vi "SR830 Read Channels.vi"(8 "error in (no error)":errorcluster caption="Error in (no error)", 10 "830?":bool, 11 "VISA Resource Name":refnum<visa-resource-name>) -> (0 "error out":errorcluster caption="Error", 1 "output2":dbl format="%#_12g", 2 "output1":dbl format="%#_12g", 3 "VISA resource name out":refnum<visa-resource-name>)   [LabVIEW 2017, in "SR830.lvlib"]
doc: "Reads the values currently displayed on the front panel of the lock-in detector."
uses:
  SR830.lvlib
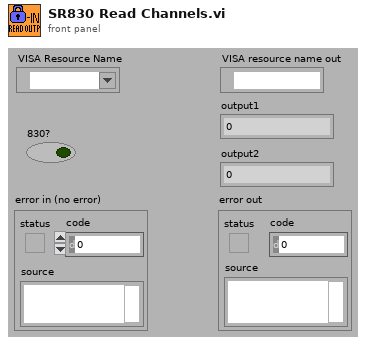
[diagram p1: front panel]
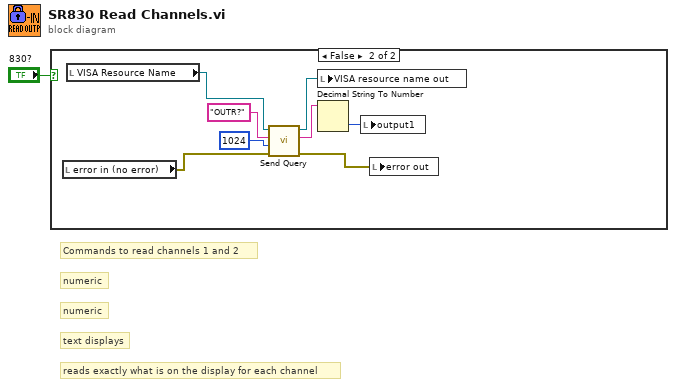
[diagram p0: block diagram]
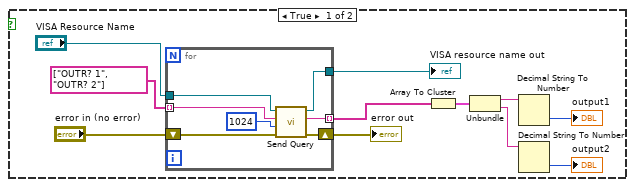
[diagram p2: hidden frame]
diagram:
  # "Commands to read channels 1 and 2"
  # "numeric"
  # "numeric"
  # "text displays"
  # "reads exactly what is on the display for each channel"
  n1 = case shown="False" "830?" {
    frame True {
      n2 = for {
        tunnel: [w15] -> w9 mode=indexing
        shift-right: [w14] -> w12
        shift-left: "error in (no error)" -> [w19]
        tunnel: "VISA Resource Name" -> [w16]
        tunnel: string[] ["OUTR? 1", "OUTR? 2"] -> [w17] mode=indexing
        tunnel: [w13] -> w6
        n3 = call "Send Query.vi"("error in (no error)"=w19, "Bytes Count"=1024, "write buffer"=w17, "VISA resource name"=w16) -> ("error out"=w14:errorcluster, "read buffer"=w15:string, "VISA resource name out"=w13:refnum<visa-resource-name>)  [unwired: 5 in]
      }
      "error out" <- w12
      "VISA resource name out" <- w6
      n4 = Array To Cluster(array=w9) -> (cluster=w10:cluster{"[0]":string, "[1]":string})
      n5 = Unbundle(w10) -> ("[0]"=w5:string, "[1]"=w4:string)
      n6 = Decimal String To Number(string=w5) -> (number=→"output1":i32)  [unwired: 2 in, 1 out]
      n7 = Decimal String To Number(string=w4) -> (number=→"output2":i32)  [unwired: 2 in, 1 out]
    }
    frame False {
      n8 = local read "error in (no error)"() -> (w21:errorcluster)
      n9 = local read "VISA Resource Name"() -> (w20:refnum<visa-resource-name>)
      n10 = call "Send Query.vi"("error in (no error)"=w21, "Bytes Count"=1024, "write buffer"="OUTR?", "VISA resource name"=w20) -> ("error out"=w25:errorcluster, "read buffer"=w23:string, "VISA resource name out"=w22:refnum<visa-resource-name>)  [unwired: 5 in]
      n11 = local write "VISA resource name out"(w22) -> ()
      n12 = Decimal String To Number(string=w23) -> (number=w26:i32)  [unwired: 2 in, 1 out]
      n13 = local write "output1"(w26) -> ()
      n14 = local write "error out"(w25) -> ()
    }
  }
